vi "Licence Activator.vi"() -> ()   [LabVIEW 2013]
panel:
  in  "generator version":string="Version: A (proto) "
  out "activation status":string="Application Dave.exe is not activated.\n\nSelect licence key file path and click Activate. If licence file is missing select licence key request file directory and click Generate Licence Key Request File. Forward the generated licence key request file to the application provider to get the licence key file."
  out "activated?":bool
  in  "licence file path":path=path "C:/LicenceKeyFile_B213D3E3-F046-42D3-9AC5-B825F6B790C1.bin"
  in  "activate/deactivate":bool
  in  "cancel":bool
  in  "generate request":bool
  in  "request file path":path=path "C:/Users/skubrick/Desktop"
  out "User name":string="Stanley Kubrick"
  out "Machine name":string="Hal 9000"
  # "Licence activation status"
  # "Licence key file path"
  # "Licence key request file directory"
  # "System informations"
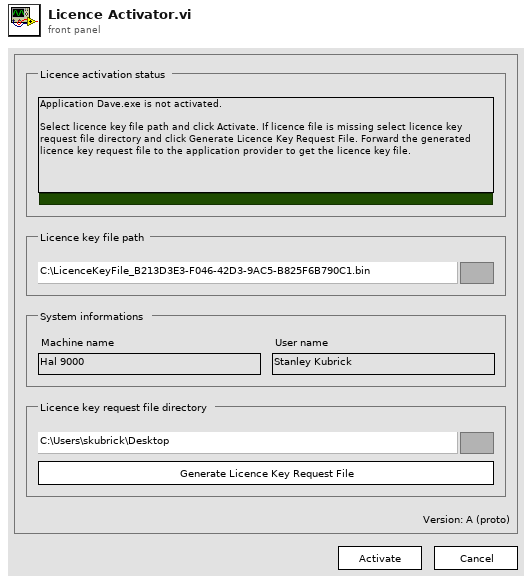
[diagram p1: front panel]
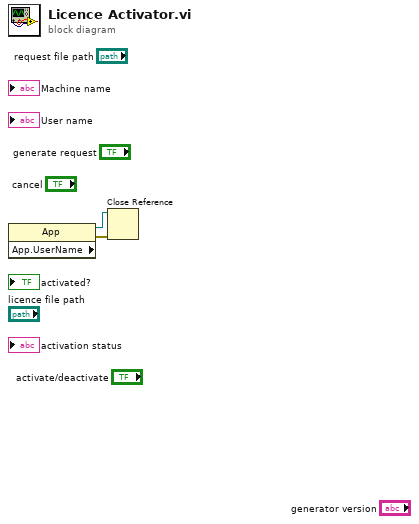
[diagram p0: block diagram]
diagram:
  n1 = property class="App" props=["App.UserName"]() -> (reference out=w1:refnum<vi>, error out=w2:errorcluster)  [unwired: 2 in, 1 out]
  n2 = Close Reference(reference=w1, error in (no error)=w2) -> ()  [unwired: 1 out]
